vi "Create Listener.vi"(8 "error in (no error)":errorcluster, 9 "timeout ms (5000)":i32=5000, 10 "Port":u16, 11 "VISA TCP Listener in":refnum<class "VISA TCP Listener.lvclass">) -> (0 "error out":errorcluster, 3 "VISA TCP Listener out":refnum<class "VISA TCP Listener.lvclass">)   [LabVIEW 2021, in "Sockets.lvlib" / "VISA TCP Listener.lvclass"]
doc: "Creates a new TCP listener on the requested port.\nWebSockets 2.0.1.40\nSam Sharp - MediaMongrels Ltd\nCopyright (c) 2019, MediaMongrels Ltd"
uses:
  VISA TCP Listener.lvclass
  VISA TCP Listener.lvclass/VISA TCP Listener.ctl
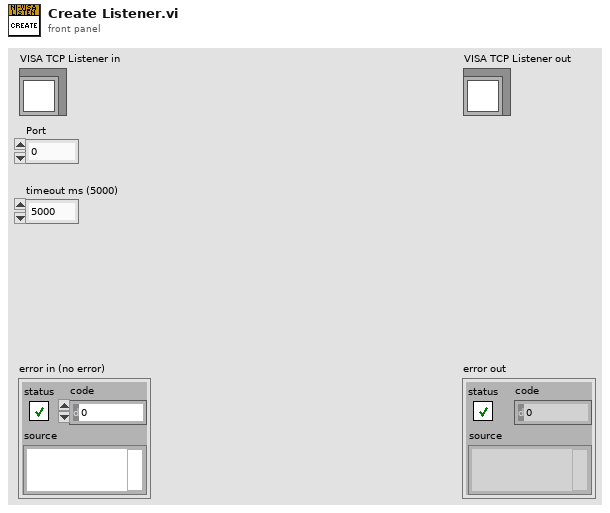
[diagram p1: front panel]
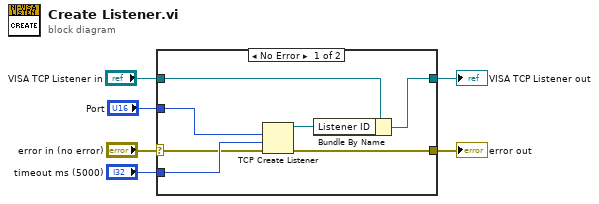
[diagram p0: block diagram]
diagram:
  n1 = case shown="No Error" "error in (no error)" {
    selector: "error in (no error)" -> [w7 w14]
    tunnel: [w13 w14] -> w6
    tunnel: "Port" -> [w12 _]
    tunnel: "timeout ms (5000)" -> [w11 _]
    tunnel: "VISA TCP Listener in" -> [w9 w15]
    tunnel: [w8 w15] -> w2
    frame No Error {
      n2 = TCP Create Listener(8:w7, 9:w11, 10:w12) -> (0:w13:errorcluster, 3:w10:refnum<k5>)  [unwired: 2 in, 1 out]
      n3 = Bundle By Name(cluster=w9, "Listener ID"=w10) -> (w8:refnum<class "VISA TCP Listener.lvclass">)
    }
    frame Error {
    }
  }
  "error out" <- w6
  "VISA TCP Listener out" <- w2
